vi "LinearMap.vi"(0 "object in":refnum<class "Utilities.lvclass">, 1 "MaxY":dbl, 5 "MaxX":dbl, 7 "X":dbl, 9 "MinX":dbl, 11 "error in (no error)":errorcluster, 12 "MinY":dbl) -> (4 "object out":refnum<class "Utilities.lvclass">, 8 "Y":dbl, 15 "error out":errorcluster)   [LabVIEW 2023, in "Utilities.lvclass"]
uses:
  Utilities.lvclass
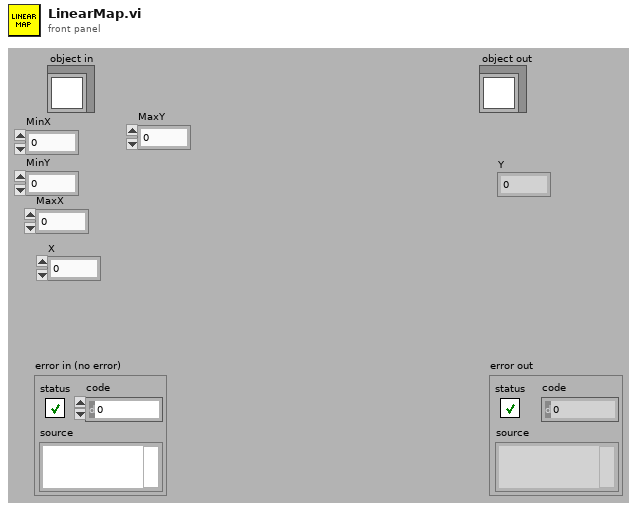
[diagram p1: front panel]
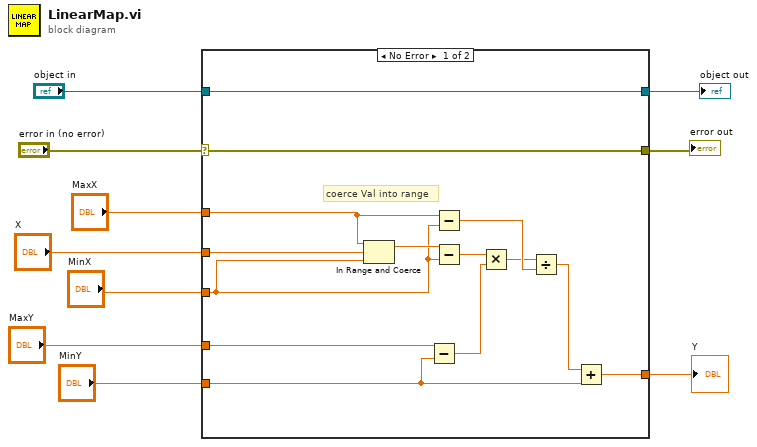
[diagram p0: block diagram]
diagram:
  n1 = case shown="No Error" "error in (no error)" {
    selector: "error in (no error)" -> [w24 w26]
    tunnel: [w24 w26] -> w9
    tunnel: [w23 w25] -> w7
    tunnel: "object in" -> [w23 w25]
    tunnel: "MinY" -> [w16 _]
    tunnel: "MaxY" -> [w12 _]
    tunnel: "X" -> [w15 _]
    tunnel: "MinX" -> [w13 _]
    tunnel: "MaxX" -> [w14 _]
    tunnel: [w11 _] -> w1
    frame No Error {
      # "coerce Val into range"
      n2 = In Range and Coerce(upper limit=w14, x=w15, lower limit=w13) -> (coerced(x)=w22:dbl)  [unwired: 1 out]
      n3 = Subtract(x=w12, y=w16) -> (x-y=w17:dbl)
      n4 = Subtract(x=w14, y=w13) -> (x-y=w20:dbl)
      n5 = Subtract(x=w22, y=w13) -> (x-y=w18:dbl)
      n6 = Multiply(x=w18, y=w17) -> (x*y=w19:dbl)
      n7 = Divide(x=w19, y=w20) -> (x/y=w21:dbl)
      n8 = Add(x=w21, y=w16) -> (x+y=w11:dbl)
    }
    frame Error {
    }
  }
  "error out" <- w9
  "object out" <- w7
  "Y" <- w1
